vi "ma_SML Filtered Spectrum by Spec.vi"(0 "spectrum properties":T1={"f0"=0.0, "df"=1.0, "#spectral lines"=0} {"df" format="%.2f"; "f0" format="%.2f"}, 1 "reset? (T)":bool=TRUE, 5 "spectral info":T3 {"window" items=["Rectangle"=0, "Hanning"=1, "Hamming"=2, "Blackman-Harris"=3, "Exact Blackman"=4, "Blackman"=5, "Flat Top"=6, "4 Term B-Harris "=7, "7 Term B-Harris"=8, "Low Sidelobe"=9, "Blackman Nuttall"=11, "Triangle"=30, "Bartlett-Hanning"=31, "Bohman"=32, "Parzen"=33, "Welch"=34, "Kaiser"=60, "Dolph-Chebyshev"=61, "Gaussian"=62]}, 7 "center channel specification":cluster{"center frequency":dbl, "bandwidth":dbl}, 9 "Adjacent Channel Specifications":cluster{"offset":dbl, "bandwidth":dbl}[](array[cluster]), 11 "error in (no error)":errorcluster, 12 "Filter Type":u16[](array[ring]) items=["None", "RRC"], 13 "Filter Parameter":dbl[](array[numeric])) -> (4 "filtered power spectrum":T2 {"spectrum" format="%.2f"; "df" format="%.2f"; "f0" format="%.2f"}, 15 "error out":errorcluster)   [LabVIEW 2020, in "NI_MAPro.lvlib"]
uses:
  NI_MAPro.lvlib
  ma_sml_Spectral Info.ctl
  ma_sml_Spectrum Cluster (real).ctl
  ma_sml_Filter Info.ctl
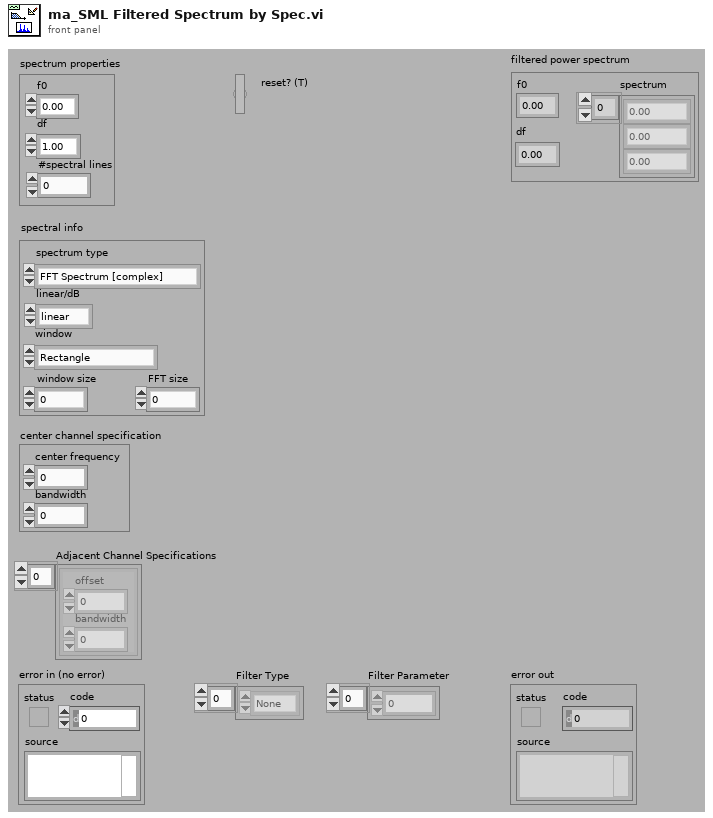
[diagram p1: front panel]
types:
  T1 = cluster{"f0":dbl, "df":dbl, "#spectral lines":i32}
  T2 = typedef "NI_MAPro.lvlib/ma_sml_Spectrum Cluster (real).ctl" = cluster{"f0":dbl, "df":dbl, "spectrum":dbl[]}
  T3 = typedef "NI_MAPro.lvlib/ma_sml_Spectral Info.ctl" = cluster{"spectrum type":enum16{"FFT Spectrum [complex]", "Amplitude [Magnitude]", "Power [Magnitude^2]", "Cross Spectrum [complex]", "Frequency Response [Complex]"}, "linear/dB":enum16{"linear", "dB"}, "window":u16, "window size":i32, "FFT size":i32}
  T4 = typedef "NI_MAPro.lvlib/ma_sml_Filter Info.ctl" = cluster{"filter type":u16, "filter parameter":dbl}
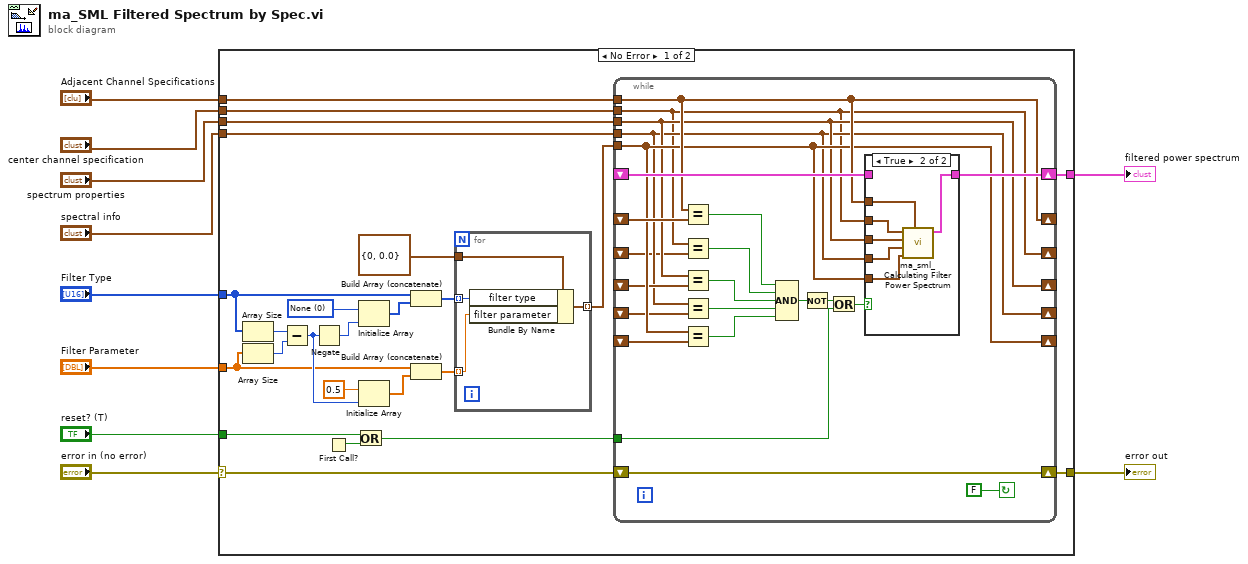
[diagram p0: block diagram]
diagram:
  n1 = case shown="No Error" "error in (no error)" {
    selector: "error in (no error)" -> [w29 w69]
    tunnel: "Adjacent Channel Specifications" -> [w34 _]
    tunnel: "center channel specification" -> [w33 _]
    tunnel: "spectral info" -> [w32 _]
    tunnel: [w28 w69] -> w8
    tunnel: "spectrum properties" -> [w30 _]
    tunnel: [w31 _] -> w6
    tunnel: "Filter Type" -> [w14 _]
    tunnel: "Filter Parameter" -> [w13 _]
    tunnel: "reset? (T)" -> [w26 _]
    frame No Error {
      w11 = u16 0 items=["None", "RRC"] ("filter type")
      n2 = Array Size(array=w14) -> (size(s)=w23:i32)
      n3 = Array Size(array=w13) -> (size(s)=w24:i32)
      n4 = Subtract(x=w23, y=w24) -> (x-y=w20:i32)
      n5 = Negate(x=w20) -> (-x=w21:i32)
      n6 = First Call?() -> (First Call?: T/F=w27:bool)
      n7 = Or(x=w26, y=w27) -> (x .or. y?=w25:bool)
      n8 = Initialize Array(w11, w21) -> (w22:u16[])
      n9 = Initialize Array(0.5 ("filter parameter"), w20) -> (w18:dbl[])
      n10 = Build Array (concatenate)(w14, w22) -> (w16:u16[])
      n11 = Build Array (concatenate)(w13, w18) -> (w17:dbl[])
      n12 = for {
        tunnel: w17 -> [w38] mode=indexing
        tunnel: w16 -> [w37] mode=indexing
        tunnel: T4 {"filter type"=0, "filter parameter"=0.0} ("pulse shaping filter") -> [w36]
        tunnel: [w35] -> w15 mode=indexing
        n13 = Bundle By Name(cluster=w36, "filter type"=w37, "filter parameter"=w38) -> (w35:T4)
      }
      n14 = while {
        tunnel: w34 -> [w57]
        tunnel: w33 -> [w45]
        tunnel: w32 -> [w51]
        tunnel: w30 -> [w52]
        tunnel: w15 -> [w54]
        shift-right: [w59] -> w28
        shift-left: w29 -> [w59]
        shift-right: [w57] -> _
        shift-left: _ -> [w56]
        shift-right: [w61] -> w31
        shift-left: _ -> [w58]
        shift-right: [w45] -> _
        shift-left: _ -> [w44]
        shift-right: [w54] -> _
        shift-left: _ -> [w55]
        shift-right: [w52] -> _
        shift-left: _ -> [w53]
        shift-right: [w51] -> _
        shift-left: _ -> [w50]
        tunnel: w25 -> [w47]
        stop <- FALSE continue-if-true
        n15 = Equal?(x=w57, y=w56) -> (x = y?=w43:bool)
        n16 = Equal?(x=w45, y=w44) -> (x = y?=w42:bool)
        n17 = Equal?(x=w52, y=w53) -> (x = y?=w41:bool)
        n18 = Equal?(x=w51, y=w50) -> (x = y?=w40:bool)
        n19 = Equal?(x=w54, y=w55) -> (x = y?=w39:bool)
        n20 = Compound Arithmetic op=AND(w43, w42, w41, w40, w39) -> (w49:bool)
        n21 = Not(x=w49) -> (.not. x?=w48:bool)
        n22 = Or(x=w48, y=w47) -> (x .or. y?=w46:bool)
        n23 = case shown="True" w46 {
          tunnel: w57 -> [_ w65]
          tunnel: w45 -> [_ w66]
          tunnel: w51 -> [_ w68]
          tunnel: [w62 w63] -> w61
          tunnel: w52 -> [_ w64]
          tunnel: w54 -> [_ w67]
          tunnel: w58 -> [w62 _]
          frame False {
          }
          frame True {
            n24 = call "ma_sml_Calculating Filter Power Spectrum.vi"("adjacent channel specifications"=w65, "filter info"=w67, "spectral info"=w68, "spectrum properties"=w64, "center channel specification"=w66) -> ("filtered power spectrum"=w63:T2)  [unwired: 6 in]
          }
        }
      }
    }
    frame Error {
    }
  }
  "filtered power spectrum" <- w6
  "error out" <- w8
